vi "Update HW Configuration File Dependency.vi"(8 "error in (no error)":errorcluster, 10 "Node Ptr dup":T1 format="%.0x", 11 "selected path in":path) -> (0 "error out":errorcluster)   [LabVIEW 2020, in "Ballard 1553 System Explorer.lvlib"]
uses:
  Ballard 1553 System Explorer.lvlib
  <vilib>/NI VeriStand/Custom Device API/Custom Device Item Ref.ctl
  <vilib>/NI VeriStand/Custom Device API/Custom Device File Dependency.ctl
  <vilib>/NI VeriStand/Custom Device API/Path Specification.ctl
  <vilib>/NI VeriStand/Custom Device API/Path Type.ctl
  <vilib>/NI VeriStand/Custom Device API/Custom Device Supported Target.ctl
  Shared/Controls and Global/Global.vi
  <vilib>/NI VeriStand/Custom Device API/Get Item Property (I32).vi
  <vilib>/NI VeriStand/Custom Device API/Custom Device API.lvlib
  Shared/Ballard 1553 Shared.lvlib
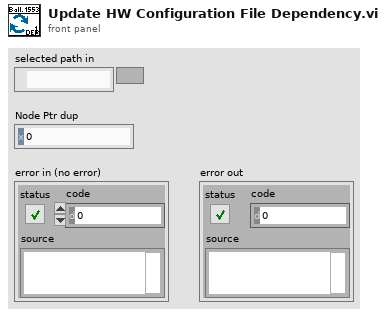
[diagram p1: front panel]
types:
  T1 = typedef "Custom Device API.lvlib/Custom Device Item Ref.ctl" = u64
  T2 = typedef "Custom Device API.lvlib/Custom Device Supported Target.ctl" = enum16{"All", "PharLap", "VxWorks", "Windows", "Linux_32_ARM", "Linux_x64", "PharLap & Windows", "PharLap & VxWorks", "VxWorks & Windows"}
  T3 = typedef "Custom Device API.lvlib/Custom Device File Dependency.ctl" = cluster{"Source":T4, "RT Destination":path, "ForceDownload?":bool, "SupportedTarget":T2, "Version":string}
  T4 = typedef "Custom Device API.lvlib/Path Specification.ctl" = cluster{"Path":path, "Type":T5}
  T5 = typedef "Custom Device API.lvlib/Path Type.ctl" = enum16{"Absolute", "To Base", "To Common Data Dir", "To Application Data Dir"}
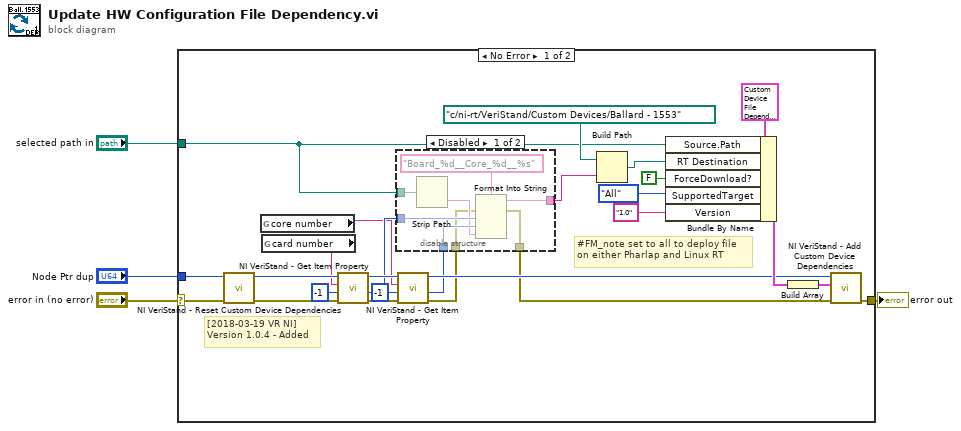
[diagram p0: block diagram]
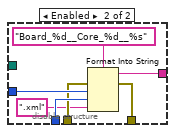
[diagram p2: hidden frame]
diagram:
  n1 = case shown="No Error" "error in (no error)" {
    selector: "error in (no error)" -> [w19 w46]
    tunnel: "Node Ptr dup" -> [w30 _]
    tunnel: "selected path in" -> [w28 _]
    tunnel: [w27 w46] -> w2
    frame No Error {
      # "#FM_note set to all to deploy file\non either Pharlap and Linux RT"
      # "[2018-03-19 VR NI]\nVersion 1.0.4 - Added"
      n2 = call <vilib>:"NI VeriStand - Reset Custom Device Dependencies.vi"("error in (no error)"=w19, "Device Ref in"=w30) -> ("error out"=w15:errorcluster, "Device Ref out"=w16:T1)  [unwired: 8 in]
      n3 = global read "Global.vi" "core number"() -> (w6:string)
      n4 = global read "Global.vi" "card number"() -> (w5:string)
      n5 = call-poly <vilib>:"NI VeriStand - Get Item Property.vi"("error in (no error)"=w15, "Default Value"=-1, "Property Name"=w5, "Item Ref in"=w16) -> ("error out"=w18:errorcluster, "Value"=w13:i32, "Item Ref out"=w17:T1)  [unwired: 4 in, 1 out]
      n6 = call-poly <vilib>:"NI VeriStand - Get Item Property.vi"("error in (no error)"=w18, "Default Value"=-1, "Property Name"=w6, "Item Ref in"=w17) -> ("error out"=w10:errorcluster, "Value"=w12:i32, "Item Ref out"=w14:T1)  [unwired: 4 in, 1 out]
      n7 = disable-structure shown="Disabled" {
        disable-tunnel: w28 -> [w38 _]
        disable-tunnel: w13 -> [w37 w45]
        disable-tunnel: w12 -> [w36 w44]
        disable-tunnel: [w34 w43] -> w11
        disable-tunnel: w10 -> [w32 w41]
        disable-tunnel: [w31 w40] -> w9
        frame Disabled {
          n8 = Strip Path(path=w38) -> (name=w35:string)  [unwired: 1 out]
          n9 = Format Into String(format string="Board_%d__Core_%d__%s", error in=w32, w37, w36, w35) -> (resulting string=w34:string, error out=w31:errorcluster)  [unwired: 1 in]
        }
        frame Enabled {
          n10 = Format Into String(format string="Board_%d__Core_%d__%s", error in=w41, w45, w44, ".xml" ("input 3")) -> (resulting string=w43:string, error out=w40:errorcluster)  [unwired: 1 in]
        }
      }
      n11 = Build Path(base path=path "c:/ni-rt/VeriStand/Custom Devices/Ballard - 1553" ("RT Destination"), name or relative path=w11) -> (appended path=w20:path)
      n12 = Bundle By Name(cluster=T3 {"Source"={"Path"=path "", "Type"=enum."Absolute"}, "RT Destination"=path "", "ForceDownload?"=FALSE, "SupportedTarget"=enum."PharLap", "Version"=""} ("Dependency"), "Source.Path"=w28, "RT Destination"=w20, "ForceDownload?"=FALSE, "SupportedTarget"=Custom_Device_Supported_Target."All", "Version"="1.0") -> (w21:T3)
      n13 = Build Array(w21) -> (w22:T3[])
      n14 = call <vilib>:"NI VeriStand - Add Custom Device Dependencies.vi"("error in (no error)"=w9, "Dependencies"=w22, "Device Ref in"=w14) -> ("error out"=w27:errorcluster)  [unwired: 7 in, 1 out]
    }
    frame Error {
    }
  }
  "error out" <- w2
